vi "rspvtd_Msg_ToServer_7.vi"(8 "error in":errorcluster, 11 "Data in":variant) -> (0 "error out":errorcluster, 3 "Data out":T1)   [LabVIEW 2019, in "gRPC Server (template.proto).lvlib" / "gRPC Server.lvclass"]
doc: "This VI converts variant data contained in the associated <b>Public API Response</b> message to its correct data type.\n---"
uses:
  gRPC Server.lvclass
  rsp_Msg_ToServer_7.ctl
  Generated_server/RPC Messages/w4lvgrpc_Msg_ToServer_7.ctl
  Generated_server/Generated_server.lvlib
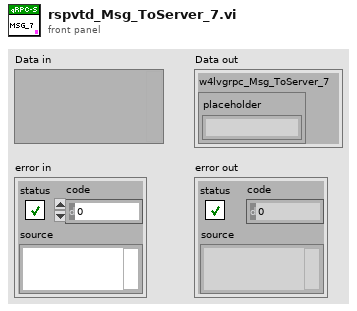
[diagram p1: front panel]
types:
  T1 = typedef "gRPC Server (template.proto).lvlib/gRPC Server.lvclass/rsp_Msg_ToServer_7.ctl" = cluster{"w4lvgrpc_Msg_ToServer_7":T2}
  T2 = typedef "Generated_server.lvlib/w4lvgrpc_Msg_ToServer_7.ctl" = cluster{"placeholder":string}
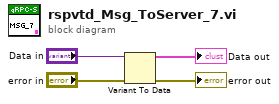
[diagram p0: block diagram]
diagram:
  n1 = Variant To Data(error in="error in", Variant="Data in") -> (data=→"Data out":T1, error out=→"error out":errorcluster)  [unwired: 1 in]
